vi "Relay Data.vi"   [LabVIEW 2013]
doc: "This VI relays information to the simulator."
uses:
  Global Variables.vi
panel:
  # "This VI relays information to the AFM simulation."
types:
  T1 = cluster{"Image Height":dbl, "Image Width":dbl, "X Offset":dbl, "Y Offset":dbl}
  T2 = cluster{"Old Image Height":dbl, "Old Image Width":dbl, "Old X Offset":dbl, "Old Y Offset":dbl}
  T3 = cluster{"Old X":dbl, "Old Y":dbl, "Old Voltage":dbl, "Old Wire Width":dbl, "Old Center of Vision":string, "Old Visible":bool, "Old RGB Value":u32}
  T4 = cluster{"X":dbl, "Y":dbl, "Voltage":dbl, "Wire Width":dbl, "Center of Vision":string, "Visible":bool, "RGB Value":u32}
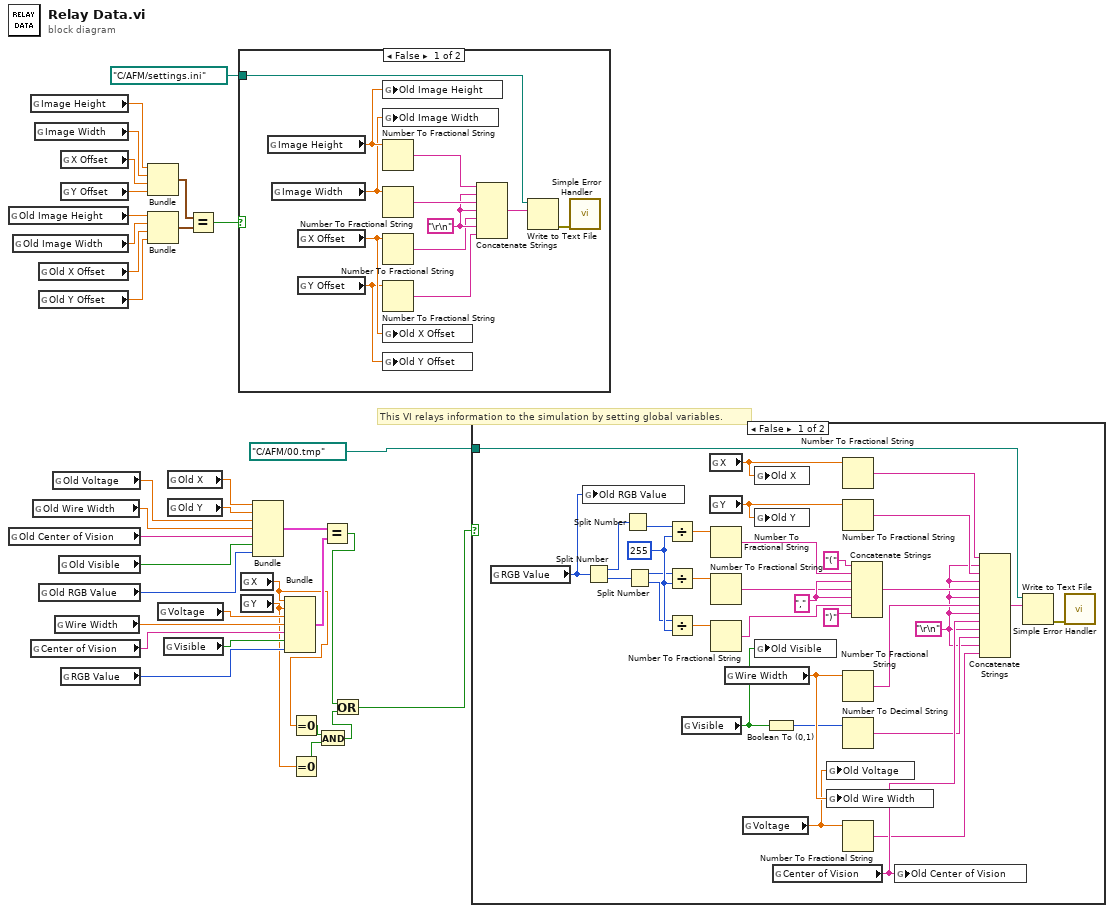
[diagram p0: block diagram]
diagram:
  # "This VI relays information to the simulation by setting global variables."
  n1 = global read "Global Variables.vi" "Old Image Height"() -> (w16:dbl)
  n2 = global read "Global Variables.vi" "Old Center of Vision"() -> (w30:string)
  n3 = global read "Global Variables.vi" "Old Image Width"() -> (w15:dbl)
  n4 = global read "Global Variables.vi" "Image Height"() -> (w20:dbl)
  n5 = global read "Global Variables.vi" "Center of Vision"() -> (w26:string)
  n6 = global read "Global Variables.vi" "Old Wire Width"() -> (w31:dbl)
  n7 = global read "Global Variables.vi" "Image Width"() -> (w19:dbl)
  n8 = global read "Global Variables.vi" "Old X Offset"() -> (w14:dbl)
  n9 = global read "Global Variables.vi" "Old Y Offset"() -> (w13:dbl)
  n10 = global read "Global Variables.vi" "Old RGB Value"() -> (w22:u32)
  n11 = global read "Global Variables.vi" "Old Voltage"() -> (w32:dbl)
  n12 = global read "Global Variables.vi" "Wire Width"() -> (w27:dbl)
  n13 = global read "Global Variables.vi" "Old Visible"() -> (w29:bool)
  n14 = global read "Global Variables.vi" "X Offset"() -> (w18:dbl)
  n15 = global read "Global Variables.vi" "Y Offset"() -> (w17:dbl)
  n16 = global read "Global Variables.vi" "RGB Value"() -> (w21:u32)
  n17 = Bundle("Image Height"=w20, "Image Width"=w19, "X Offset"=w18, "Y Offset"=w17) -> (w12:T1)  [unwired: 1 in]
  n18 = Bundle("Old Image Height"=w16, "Old Image Width"=w15, "Old X Offset"=w14, "Old Y Offset"=w13) -> (w11:T2)  [unwired: 1 in]
  n19 = global read "Global Variables.vi" "Voltage"() -> (w28:dbl)
  n20 = global read "Global Variables.vi" "Visible"() -> (w25:bool)
  n21 = global read "Global Variables.vi" "Old X"() -> (w34:dbl)
  n22 = global read "Global Variables.vi" "Old Y"() -> (w33:dbl)
  n23 = Equal?(x=w12, y=w11) -> (x = y?=w10:bool)
  n24 = case shown="False" w10 {
    tunnel: path "C:/AFM/settings.ini" ("base path") -> [w42 _]
    frame False {
      w39 = "\r\n"
      n25 = global read "Global Variables.vi" "Image Height"() -> (w41:dbl)
      n26 = global read "Global Variables.vi" "Image Width"() -> (w40:dbl)
      n27 = global read "Global Variables.vi" "X Offset"() -> (w38:dbl)
      n28 = global read "Global Variables.vi" "Y Offset"() -> (w37:dbl)
      n29 = global write "Global Variables.vi" "Old Image Height"(w41) -> ()
      n30 = global write "Global Variables.vi" "Old Image Width"(w40) -> ()
      n31 = Number To Fractional String(number=w41) -> (F-format string=w46:string)  [unwired: 3 in]
      n32 = Number To Fractional String(number=w40) -> (F-format string=w45:string)  [unwired: 3 in]
      n33 = Number To Fractional String(number=w38) -> (F-format string=w36:string)  [unwired: 3 in]
      n34 = Number To Fractional String(number=w37) -> (F-format string=w35:string)  [unwired: 3 in]
      n35 = global write "Global Variables.vi" "Old X Offset"(w38) -> ()
      n36 = global write "Global Variables.vi" "Old Y Offset"(w37) -> ()
      n37 = Concatenate Strings(w46, w39, w45, w39, w36, w39, w35) -> (w44:string)
      n38 = Write to Text File(file (use dialog)=w42, text=w44) -> (error out=w43:errorcluster)  [unwired: 2 in, 2 out]
      n39 = call <vilib>:"Simple Error Handler.vi"("error in (no error)"=w43) -> ()  [unwired: 4 in, 5 out]
    }
    frame True {
    }
  }
  n40 = global read "Global Variables.vi" "X"() -> (w7:dbl)
  n41 = global read "Global Variables.vi" "Y"() -> (w6:dbl)
  n42 = Bundle("Old X"=w34, "Old Y"=w33, "Old Voltage"=w32, "Old Wire Width"=w31, "Old Center of Vision"=w30, "Old Visible"=w29, "Old RGB Value"=w22) -> (w24:T3)  [unwired: 1 in]
  n43 = Bundle("X"=w7, "Y"=w6, "Voltage"=w28, "Wire Width"=w27, "Center of Vision"=w26, "Visible"=w25, "RGB Value"=w21) -> (w23:T4)  [unwired: 1 in]
  n44 = Equal To 0?(x=w7) -> (x = 0?=w5:bool)
  n45 = Equal To 0?(x=w6) -> (x = 0?=w4:bool)
  n46 = And(x=w5, y=w4) -> (x .and. y?=w3:bool)
  n47 = Equal?(x=w24, y=w23) -> (x = y?=w2:bool)
  n48 = Or(x=w2, y=w3) -> (x .or. y?=w1:bool)
  n49 = case shown="False" w1 {
    tunnel: path "C:/AFM/00.tmp" ("file (use dialog)") -> [w75 _]
    frame False {
      w58 = u8 255 ("y")
      w63 = "," ("string")
      w55 = "\r\n"
      n50 = global read "Global Variables.vi" "RGB Value"() -> (w47:u32)
      n51 = global write "Global Variables.vi" "Old RGB Value"(w47) -> ()
      n52 = Split Number(x=w47) -> (hi(x)=w52:u16, lo(x)=w53:u16)
      n53 = Split Number(x=w52) -> (lo(x)=w50:u8)  [unwired: 1 out]
      n54 = Split Number(x=w53) -> (hi(x)=w49:u8, lo(x)=w48:u8)
      n55 = Divide(x=w50, y=w58) -> (x/y=w59:dbl)
      n56 = Divide(x=w49, y=w58) -> (x/y=w56:dbl)
      n57 = Divide(x=w48, y=w58) -> (x/y=w57:dbl)
      n58 = global read "Global Variables.vi" "Visible"() -> (w69:bool)
      n59 = global read "Global Variables.vi" "X"() -> (w74:dbl)
      n60 = global read "Global Variables.vi" "Y"() -> (w73:dbl)
      n61 = Number To Fractional String(number=w59) -> (F-format string=w64:string)  [unwired: 3 in]
      n62 = Number To Fractional String(number=w56) -> (F-format string=w62:string)  [unwired: 3 in]
      n63 = Number To Fractional String(number=w57) -> (F-format string=w61:string)  [unwired: 3 in]
      n64 = global read "Global Variables.vi" "Wire Width"() -> (w72:dbl)
      n65 = global read "Global Variables.vi" "Voltage"() -> (w51:dbl)
      n66 = global write "Global Variables.vi" "Old X"(w74) -> ()
      n67 = global write "Global Variables.vi" "Old Y"(w73) -> ()
      n68 = global write "Global Variables.vi" "Old Visible"(w69) -> ()
      n69 = Boolean To (0,1)(Boolean=w69) -> (0, 1=w68:i16)
      n70 = global read "Global Variables.vi" "Center of Vision"() -> (w71:string)
      n71 = global write "Global Variables.vi" "Old Voltage"(w51) -> ()
      n72 = global write "Global Variables.vi" "Old Wire Width"(w72) -> ()
      n73 = Number To Fractional String(number=w74) -> (F-format string=w79:string)  [unwired: 3 in]
      n74 = Number To Fractional String(number=w73) -> (F-format string=w78:string)  [unwired: 3 in]
      n75 = Number To Fractional String(number=w72) -> (F-format string=w70:string)  [unwired: 3 in]
      n76 = Number To Decimal String(number=w68) -> (decimal integer string=w67:string)  [unwired: 1 in]
      n77 = Number To Fractional String(number=w51) -> (F-format string=w54:string)  [unwired: 3 in]
      n78 = Concatenate Strings("(" ("string"), w64, w63, w62, w63, w61, ")" ("string")) -> (w66:string)
      n79 = global write "Global Variables.vi" "Old Center of Vision"(w71) -> ()
      n80 = Concatenate Strings(w79, w55, w78, w55, w66, w55, w70, w55, w71, w55, w67, w55, w54) -> (w77:string)
      n81 = Write to Text File(file (use dialog)=w75, text=w77) -> (error out=w76:errorcluster)  [unwired: 2 in, 2 out]
      n82 = call <vilib>:"Simple Error Handler.vi"("error in (no error)"=w76) -> ()  [unwired: 4 in, 5 out]
    }
    frame True {
    }
  }
